vi "6.vi"() -> ()   [LabVIEW 2023]
uses:
  <vilib>/gmath/zero.llb/Find All Zeros of f(x) (Formula).vi
  <vilib>/gmath/NI_Gmath.lvlib
panel:
  out "Solutii":dbl[](array[numeric]) format="%#_2g"
  out "Mesaj":string
  out "Led":bool
  in  "Formula":string
  in  "Interval solutii":cluster{dbl, dbl}(slide)={0.0, -10.0} scale=-10.0..10.0
  in  "Stop Button":bool
  out "XY Graph":cluster{dbl[], dbl[]}[](graph)
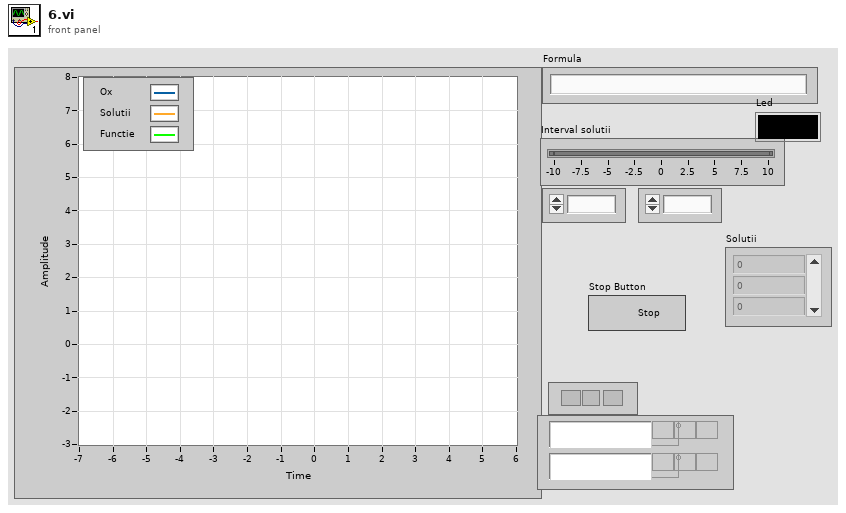
[diagram p1: front panel]
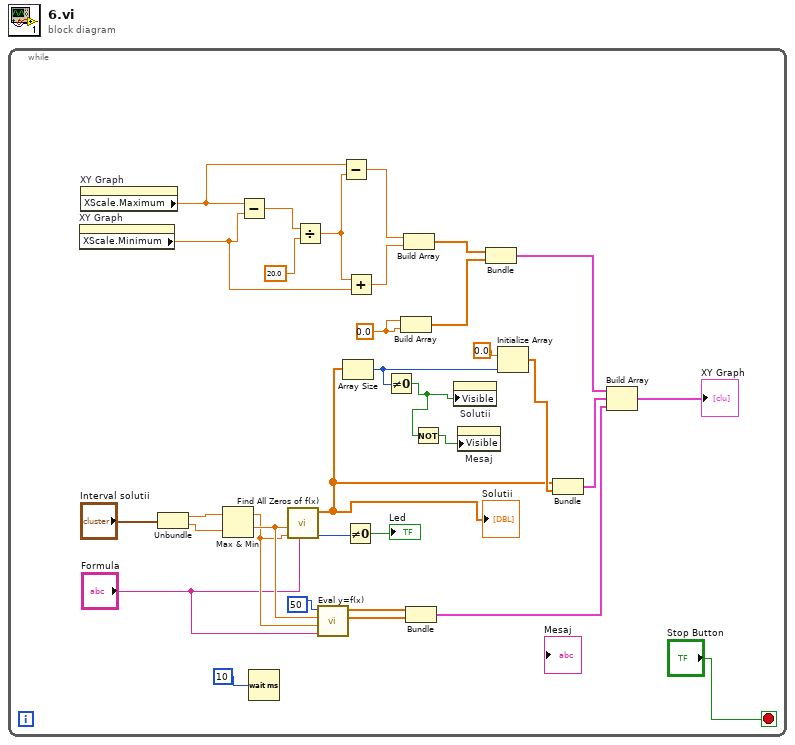
[diagram p0: block diagram]
diagram:
  n1 = while {
    stop <- "Stop Button" stop-if-true
    w26 = 0.0
    n2 = property on="XY Graph" class="XYGraph (strict)"() -> ("XScale.Minimum"=w30:dbl)  [unwired: 2 in, 2 out]
    n3 = property on="XY Graph" class="XYGraph (strict)"() -> ("XScale.Maximum"=w33:dbl)  [unwired: 2 in, 2 out]
    n4 = Unbundle "Unbundle"("Interval solutii") -> (w20:dbl, w19:dbl)
    n5 = Max & Min(x=w20, y=w19) -> (max(x,y)=w15:dbl, min(x,y)=w16:dbl)
    n6 = Subtract(x=w33, y=w30) -> (x-y=w32:dbl)
    n7 = Wait (ms)(milliseconds to wait=10) -> ()  [unwired: 1 out]
    n8 = call-poly <vilib>:"Find All Zeros of f(x).vi"("formula"="Formula", "end"=w15, "start"=w16) -> ("error"=w17:i32, "Zeros"=w2:dbl[])  [unwired: 5 in, 2 out]
    "Solutii" <- w2
    n9 = Divide(x=w32, y=20.0) -> (x/y=w29:dbl)
    n10 = call <vilib>:"Eval y=f(x).vi"("formula"="Formula", "end"=w15, "start"=w16, "number of points"=50) -> ("Y Values"=w11:dbl[], "X Values"=w12:dbl[])  [unwired: 2 out]
    n11 = Subtract(x=w33, y=w29) -> (x-y=w28:dbl)
    n12 = Array Size(array=w2) -> (size(s)=w6:i32)
    n13 = Not Equal To 0?(x=w17) -> (x != 0?=→"Led":bool)
    n14 = Add(x=w29, y=w30) -> (x+y=w27:dbl)
    n15 = Not Equal To 0?(x=w6) -> (x != 0?=w1:bool)
    n16 = Build Array "Build Array"(w26, w26) -> (w24:dbl[])
    n17 = Build Array "Build Array"(w28, w27) -> (w25:dbl[])
    n18 = Bundle "Bundle"("X Values"=w12, "Y Values"=w11) -> (w10:cluster{"X Values":dbl[], "Y Values":dbl[]})  [unwired: 1 in]
    n19 = Not(x=w1) -> (.not. x?=w5:bool)
    n20 = property on="Solutii" class="Arr (strict)"("Visible"=w1) -> ()  [unwired: 2 in, 2 out]
    n21 = property on="Mesaj" class="Str"("Visible"=w5) -> ()  [unwired: 2 in, 2 out]
    n22 = Bundle "Bundle"(w25, w24) -> (w23:cluster{dbl[], dbl[]})  [unwired: 1 in]
    n23 = Initialize Array "Initialize Array"(0.0, w6) -> (w7:dbl[])
    n24 = Bundle "Bundle"("Zeros"=w2, w7) -> (w9:cluster{"Zeros":dbl[], dbl[]})  [unwired: 1 in]
    n25 = Build Array(w23, w9, w10) -> (→"XY Graph":cluster{"X Values":dbl[], "Y Values":dbl[]}[])
  }
